vi "Add Module.vi"(8 "error in (no error)":errorcluster, 10 "Module path":string, 11 ".NET Refnum in":refnum<k24>) -> (0 "error out":errorcluster, 2 "Unique module identifier":string, 3 ".NET Refnum out":refnum<k24>)   [LabVIEW 2017, in "Routing and Faulting Scripting.lvlib"]
uses:
  Routing and Faulting Scripting.lvlib
  NationalInstruments.VeriStand.SystemStorage
  Constants/Scripting Constants.vi
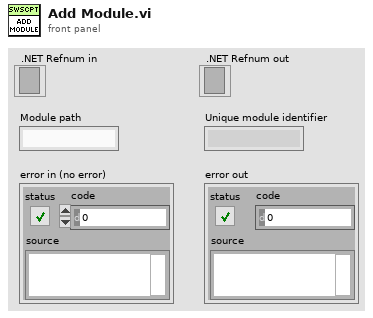
[diagram p1: front panel]
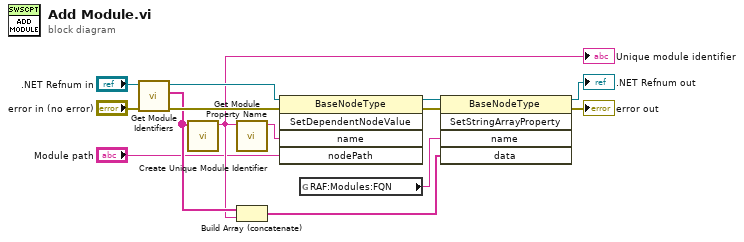
[diagram p0: block diagram]
diagram:
  n1 = call "Get Module Identifiers.vi"("error in (no error)"="error in (no error)", ".NET Refnum in"=".NET Refnum in") -> ("error out"=w13:errorcluster, "Module Identifier"=w10:string[], ".NET Refnum out"=w14:refnum<k24>)  [unwired: 7 in]
  n2 = call "Create Unique Module Identifier.vi"("Existing Module Identifiers"=w10) -> ("Unique Module Identifier"=w7:string)  [unwired: 10 in]
  "Unique module identifier" <- w7
  n3 = call "Get Module Property Name.vi"("Module ID"=w7) -> ("Module Property Name"=w2:string)  [unwired: 10 in]
  n4 = Build Array (concatenate)(w10, w7) -> (w6:string[])
  n5 = invoke class="BaseNodeType" method="SetDependentNodeValue"(reference=w14, error in=w13, "name"=w2, "nodePath"="Module path") -> (reference out=w3:refnum<k24>, error out=w5:errorcluster)  [unwired: 1 in, 3 out]
  n6 = global read "Scripting Constants.vi" "RAF:Modules:FQN"() -> (w9:string)
  n7 = invoke class="BaseNodeType" method="SetStringArrayProperty"(reference=w3, error in=w5, "name"=w9, "data"=w6) -> (reference out=→".NET Refnum out":refnum<k24>, error out=→"error out":errorcluster)  [unwired: 1 in, 3 out]
